vi "IRH3T_FIFO.vi"(8 "Due Dates":u16[](array[numeric]), 9 "Initial Tardiness":u16, 10 "Schedule 2B Improved":u16[](array[numeric]), 11 "Proocessing Times  (Machines x Jobs)":u16[][](array[numeric])=[[208, 80, 8, 184, 218, 197, 100, 5], [64, 30, 39, 91, 257, 38, 34, 447], [23, 215, 125, 135, 165, 136, 164, 37], [88, 22, 207, 5, 58, 213, 52, 355], [6, 181, 111, 222, 27, 259, 91, 103], [149, 37, 22, 14, 71, 155, 536, 16], [113, 71, 274, 348, 187, 1, 3, 3], [349, 364, 214, 1, 17, 1, 20, 34]]) -> (1 "IRH3T Schedule Out":u16[](array[numeric]), 2 "Total Tardiness":i32, 3 "IRH3T (Reordered) Schedule Out":u16[](array[numeric]))   [LabVIEW 2013]
uses:
  Classes/GanntChart_Class/Check Other Machines for Schedule Time.vi
  Classes/GanntChart_Class/Schedule Job.vi
  Classes/GanntChart_Class/Find Gaps on Particular Machine.vi
  Classes/GanntChart_Class/Increment Number of Jobs on Machine.vi
  Classes/GanntChart_Class/Operation to Machine Job Tuple.vi
  Classes/GanntChart_Class/Find Job On Other Machines.vi
  Classes/GanntChart.lvclass
panel:
  out "String":string="Total Tardiness has been improved. Total Tardiness is now %d"
  out "Job Completion Times":u16[](array[numeric])
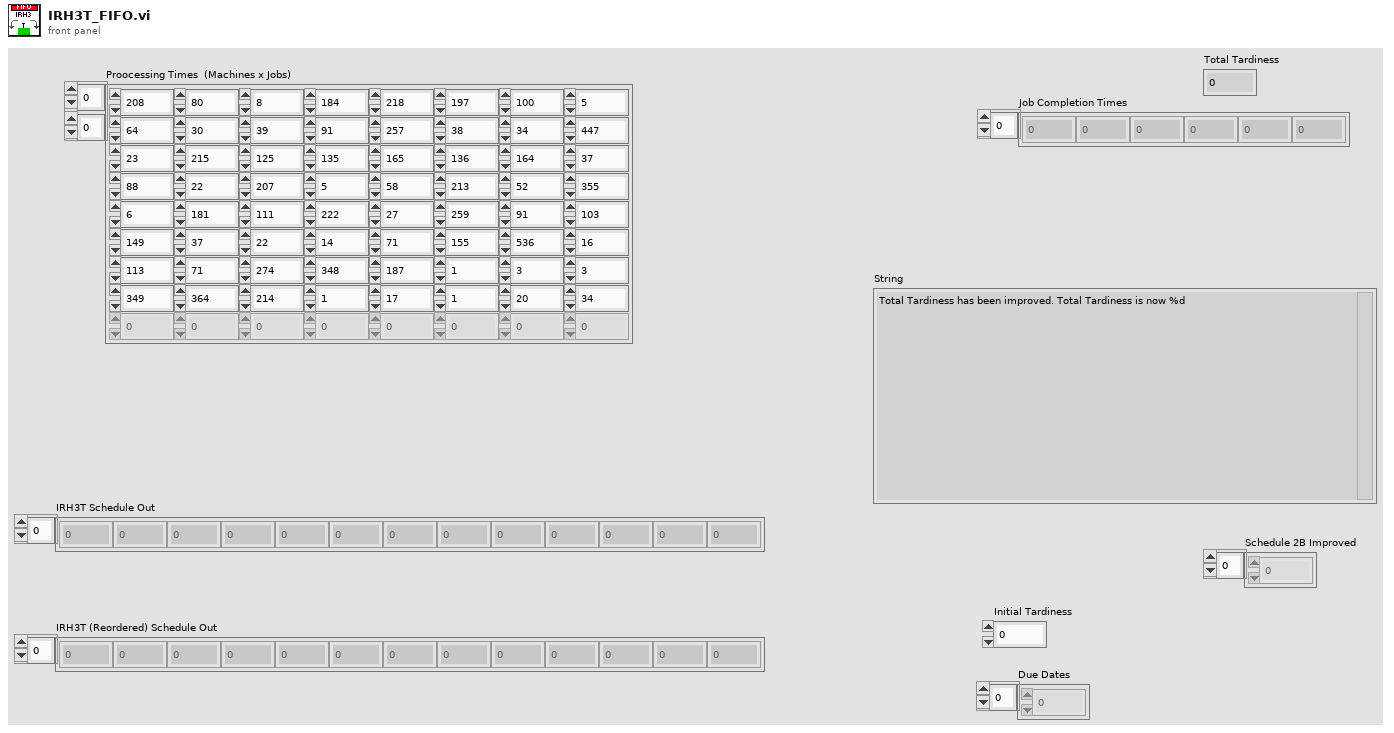
[diagram p1: front panel]
types:
  T1 = typedef "GanntChart_Element.ctl" = cluster{"Operation Number":i32, "Job Number":i32, "Start Time":i32, "Procesing Time":u16, "End Time":i32}
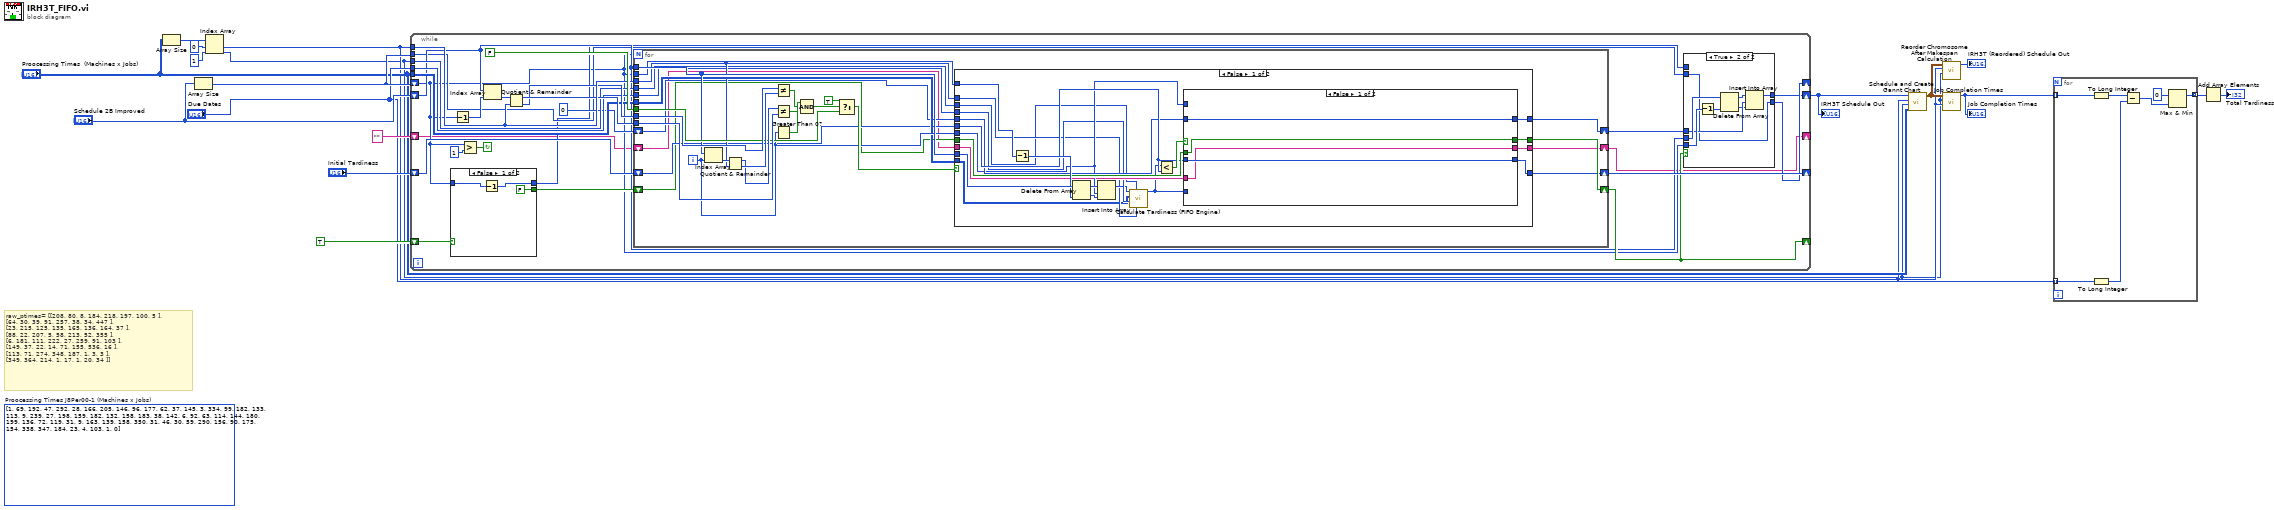
[diagram p0: block diagram]
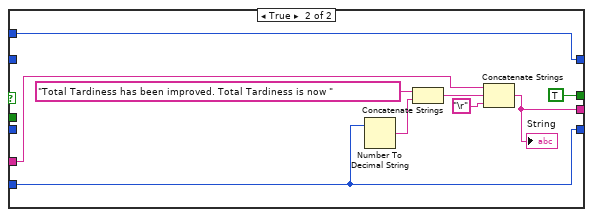
[diagram p3: hidden frame]
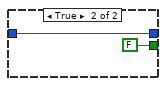
[diagram p5: hidden frame]
diagram:
  (unwired) u16[][] [[1, 69, 192, 47, 292, 28, 166, 205], [146, 96, 177, 62, 37, 145, 3, 334], [99, 182, 133, 113, 9, 239, 27, 198], [159, 182, 132, 158, 183, 38, 142, 6], [92, 63, 114, 144, 180, 199, 136, 72], [119, 31, 9, 163, 139, 158, 350, 31], [46, 30, 59, 290, 156, 90, 175, 154], [338, 347, 184, 23, 4, 103, 1, 0]]  # Proocessing Times J8Per00-1 (Machines x Jobs)
  # "raw_ptimes= [[208, 80, 8, 184, 218, 197, 100, 5 ],\n[64, 30, 39, 91, 257, 38, 34, 447 ],\n[23, 215, 125, 135, 165, 136, 164, 37 ],\n[88, 22, 207, 5, 58, 213, 52, 355 ],\n[6, 181, 111, 222, 27, 259, 91, 103 ],\n[149, 37, 22, 14, 71, 155, 536, 16 ],\n[113, 71, 274, 348, 187, 1, 3, 3 ],\n[349, 364, 214, 1, 17, 1, 20, 34 ]]"
  n1 = Array Size(array="Proocessing Times  (Machines x Jobs)") -> (size(s)=w15:i32[])
  n2 = Array Size(array="Schedule 2B Improved") -> (size(s)=w12:i32)
  n3 = Index Array(array=w15, index #1=0 ("index"), index #2=1 ("index")) -> (element #1=w3:i32, element #2=w2:i32)
  n4 = while {
    shift-right: [w24] -> _
    shift-left: w12 -> [w22]
    shift-right: [w28] -> _
    shift-left: TRUE -> [w42]
    tunnel: w3 -> [w38]
    tunnel: "Proocessing Times  (Machines x Jobs)" -> [w35]
    tunnel: w2 -> [w34]
    tunnel: "Due Dates" -> [w33]
    shift-right: [w30] -> _
    shift-left: "Initial Tardiness" -> [w32]
    shift-right: [w21] -> w7
    shift-left: "Schedule 2B Improved" -> [w27]
    tunnel: w12 -> [w25]
    shift-right: [w19] -> _
    shift-left: "" -> [w20]
    stop <- w43 continue-if-true
    n5 = case shown="False" w42 {
      tunnel: w22 -> [w122 w124]
      tunnel: [w121 w124] -> w23
      tunnel: [FALSE FALSE] -> w31
      frame False {
        n6 = Decrement(x=w122) -> (x-1=w121:i32)
      }
      frame True {
      }
    }
    n7 = Decrement(x=w22) -> (x-1=w41:i32)
    n8 = Greater?(x=w22, y=1) -> (0:w43:bool)
    n9 = Index Array(array=w27, index=w41) -> (element=w40:u16)
    n10 = Quotient & Remainder(x=w40, y=w38) -> (x-y*floor(x/y)=w37:i32, floor(x/y)=w36:i32)
    n11 = for {
      N: w22 -> [_]
      tunnel: FALSE -> [w72]
      tunnel: w27 -> [w69]
      tunnel: w38 -> [w65]
      tunnel: w37 -> [w75]
      tunnel: w36 -> [w79]
      tunnel: w22 -> [w68]
      tunnel: w35 -> [w66]
      tunnel: w34 -> [w64]
      tunnel: w33 -> [w63]
      shift-right: [w60] -> w28
      shift-left: w31 -> [w61]
      shift-right: [w59] -> w30
      shift-left: w32 -> [w62]
      shift-right: [w57] -> w26
      shift-left: 0 -> [w58]
      shift-right: [w55] -> w19
      shift-left: w20 -> [w56]
      i -> [w67]
      n12 = Index Array(array=w69, index=w67) -> (element=w81:u16)
      n13 = Quotient & Remainder(x=w81, y=w65) -> (x-y*floor(x/y)=w76:i32, floor(x/y)=w78:i32)
      n14 = Not Equal?(x=w79, y=w78) -> (x != y?=w77:bool)
      n15 = Not Equal?(x=w76, y=w75) -> (x != y?=w74:bool)
      n16 = Greater Than 0?(x=w67) -> (x > 0?=w80:bool)
      n17 = Compound Arithmetic op=AND(w80, w77, w74) -> (w73:bool)
      n18 = Select(t=TRUE, s=w73, f=w72) -> (s? t:f=w70:bool)
      n19 = case shown="False" w70 {
        tunnel: w69 -> [w102 _]
        tunnel: w68 -> [w101 _]
        tunnel: w67 -> [w91 _]
        tunnel: w66 -> [w82 _]
        tunnel: w65 -> [w84 _]
        tunnel: w64 -> [w83 _]
        tunnel: w63 -> [w86 _]
        tunnel: w62 -> [w94 w118]
        tunnel: w61 -> [w97 w119]
        tunnel: [w96 w119] -> w60
        tunnel: [w95 w118] -> w59
        tunnel: w58 -> [w93 w117]
        tunnel: [w92 w117] -> w57
        tunnel: w56 -> [w90 w116]
        tunnel: [w89 w116] -> w55
        frame False {
          n20 = Decrement(x=w101) -> (x-1=w100:i32)
          n21 = Delete From Array(array=w102, index=w100) -> (deleted portion=w88:u16, array with subset deleted=w99:u16[])  [unwired: 1 in]
          n22 = Insert Into Array(array=w99, index=w91, new element=w88) -> (w85:u16[])
          n23 = call "Calculate Tardiness (FIFO Engine).vi"("Number of Machines"=w84, "Number of Jobs"=w83, "Due Dates"=w86, "Processing Times"=w82, "Schedule In"=w85) -> ("Tardiness(FIFO Engine)"=w87:u16)  [unwired: 6 in]
          n24 = Less?(x=w87, y=w94) -> (x < y?=w98:bool)
          n25 = case shown="False" w98 {
            tunnel: [w106 TRUE] -> w96
            tunnel: w97 -> [w106 _]
            tunnel: w87 -> [_ w113]
            tunnel: [w105 w113] -> w95
            tunnel: w94 -> [w105 _]
            tunnel: w93 -> [w104 _]
            tunnel: [w104 w114] -> w92
            tunnel: w91 -> [_ w114]
            tunnel: w90 -> [w103 w110]
            tunnel: [w103 w107] -> w89
            frame False {
            }
            frame True {
              n26 = Number To Decimal String(number=w113) -> (decimal integer string=w112:string)  [unwired: 1 in]
              n27 = Concatenate Strings("Total Tardiness has been improved. Total Tardiness is now ", w112) -> (w109:string)
              n28 = Concatenate Strings(w110, w109, "\r") -> (w107:string)
              "String" <- w107
            }
          }
        }
        frame True {
        }
      }
    }
    n29 = case shown="True" w28 {
      tunnel: w27 -> [w45 w54]
      tunnel: w22 -> [_ w52]
      tunnel: w26 -> [_ w50]
      tunnel: [w46 w48] -> w24
      tunnel: w25 -> [_ w48]
      tunnel: w23 -> [w46 _]
      tunnel: [w45 w47] -> w21
      frame False {
      }
      frame True {
        n30 = Decrement(x=w52) -> (x-1=w53:i32)
        n31 = Delete From Array(array=w54, index=w53) -> (deleted portion=w49:u16, array with subset deleted=w51:u16[])  [unwired: 1 in]
        n32 = Insert Into Array(array=w51, index=w50, new element=w49) -> (w47:u16[])
      }
    }
  }
  "IRH3T Schedule Out" <- w7
  n33 = call "Schedule and Create Gannt Chart.vi"("Processing Times (Rows Mach.Cols Jobs)"="Proocessing Times  (Machines x Jobs)", "Number of Jobs"=w2, "Number of Machines"=w3, "Schedule"=w7) -> ("Gannt Chart Out"=w4:T1[][])  [unwired: 6 in, 1 out]
  n34 = call "Reorder Chromosome  After Makespan Calculation.vi"("Number Of  Jobs"=w2, "Number Of Machines"=w3, "Gannt Chart In"=w4) -> ("Reordered Chromosome"=→"IRH3T (Reordered) Schedule Out":u16[])  [unwired: 8 in]
  n35 = call "Job Completion Times.vi"("Number Of Machines"=w3, "Number Of Jobs"=w2, "Gannt Chart In"=w4) -> ("Job Completion Times"=w5:u16[])  [unwired: 8 in]
  "Job Completion Times" <- w5
  n36 = for {
    tunnel: w5 -> [w128] mode=indexing
    tunnel: "Due Dates" -> [w127] mode=indexing
    tunnel: [w129] -> w11 mode=indexing
    n37 = To Long Integer(number=w128) -> (32bit integer=w125:i32)
    n38 = To Long Integer(number=w127) -> (32bit integer=w126:i32)
    n39 = Subtract(x=w125, y=w126) -> (x-y=w131:i32)
    n40 = Max & Min(x=0, y=w131) -> (max(x,y)=w129:i32)  [unwired: 1 out]
  }
  n41 = Add Array Elements(numeric array=w11) -> (sum=→"Total Tardiness":i32)
